vi "gcn_directory_monitor.vi"() -> ()   [LabVIEW 2017]
doc: "This example shows how we can use directory change notifications within the Windows API to monitor a folder for a change in a certain directory. We utilize the FindFirstChangeNotification to set up our events to monitor. We then utilize the wait functions to trigger a LV event when a change has been made to the directory. For more information on the Windows API, visit the MSDN."
panel:
  in  "browser_link":path
  in  "WebBrowser":refnum<k7>(container)
  in  "Stop Button":bool
  in  "Added?":string
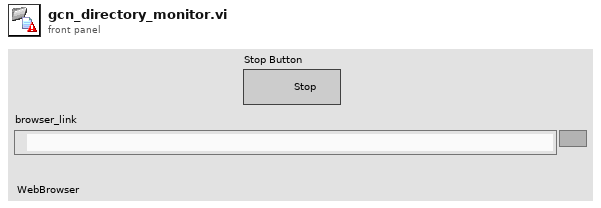
[diagram p1: front panel]
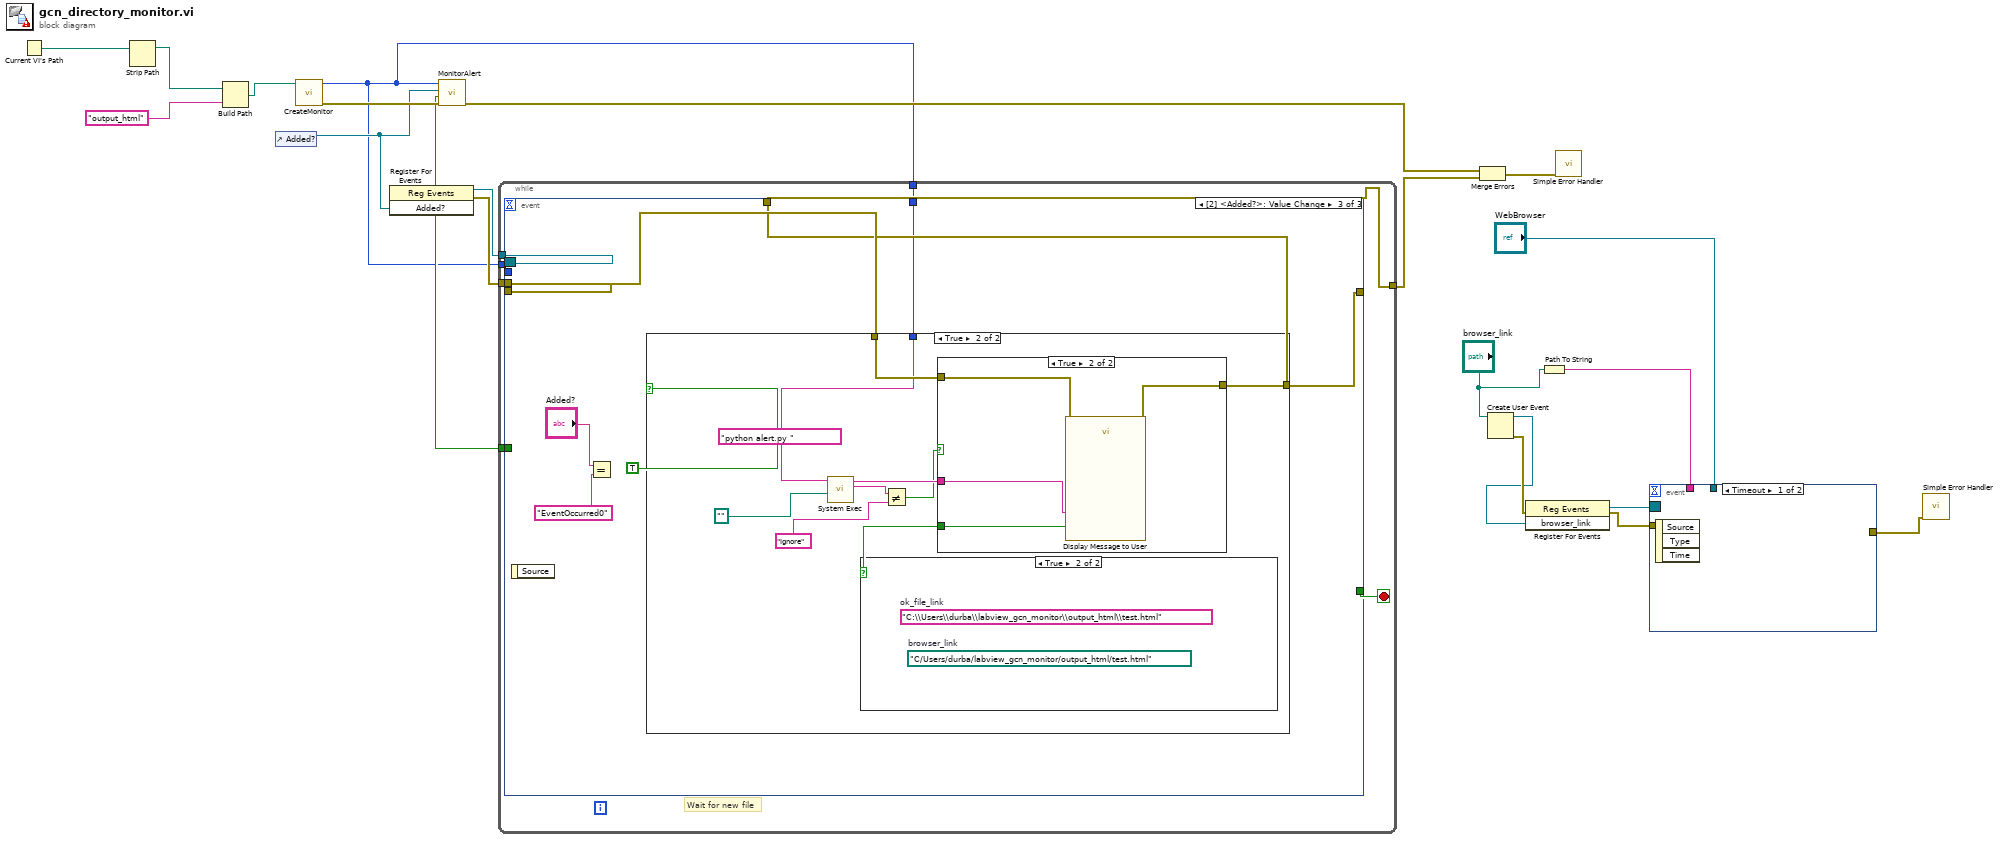
[diagram p0: block diagram]
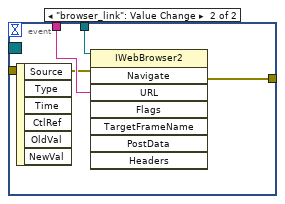
[diagram p2: hidden frame]
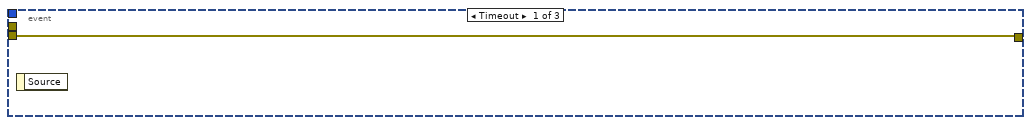
[diagram p3: hidden frame]
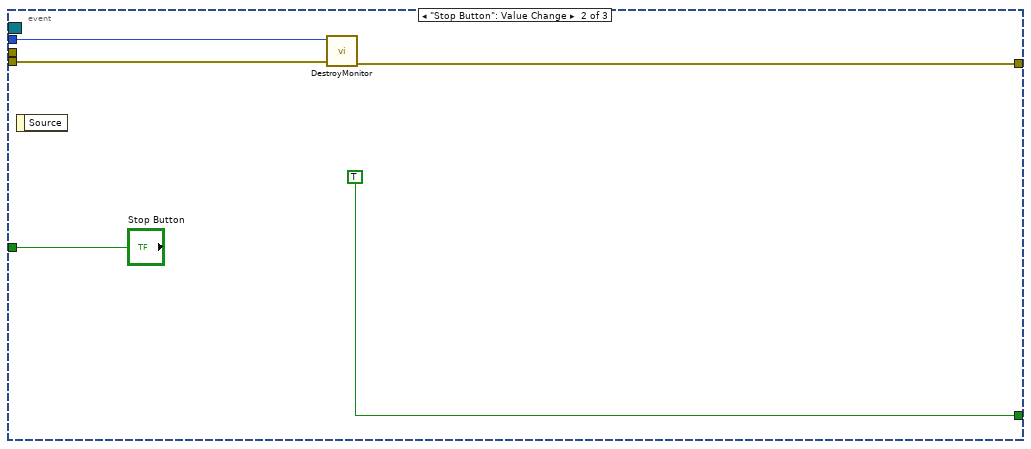
[diagram p4: hidden frame]
diagram:
  n1 = Current VI's Path() -> (path=w19:path)
  n2 = Strip Path(path=w19) -> (stripped path=w18:path)  [unwired: 1 out]
  n3 = Build Path(base path=w18, name or relative path="output_html") -> (appended path=w17:path)
  n4 = control-ref of="Added?"() -> (w20:refnum<vi>)
  n5 = call "CreateMonitor.vi"("File Path Control"=w17) -> ("error out"=w21:errorcluster, "Handle"=w1:i32)  [unwired: 9 in]
  n6 = register-events(w20) -> (reference out=w11:refnum<event-registration>, error out=w12:errorcluster)  [unwired: 2 in]
  n7 = while {
    tunnel: w1 -> [w27]
    tunnel: w11 -> [w26]
    tunnel: [w24] -> w14
    tunnel: w12 -> [w25]
    tunnel: [w23] -> w2
    tunnel: w1 -> [w22]
    stop <- w28 stop-if-true
    # "Wait for new file"
    n8 = event shown="[2] <Added?>: Value Change" {
      selector: w26 -> [_ _ _]
      dyn-events: _ -> [_ _ _]
      timeout: _ -> [_ _ _]
      tunnel: [_ TRUE _] -> w28
      tunnel: w27 -> [_ w34 _]
      tunnel: [w29 w32 w37] -> _
      tunnel: w25 -> [w29 w31 _]
      tunnel: w25 -> [_ _ w40]
      tunnel: [_ _ w37] -> w24
      tunnel: [_ "Stop Button" _] -> w23
      tunnel: w22 -> [_ _ w35]
      event Timeout {
        n9 = event-data() -> ()  [unwired: 1 in, 1 out]
      }
      event "Stop Button": Value Change {
        n10 = event-data() -> ()  [unwired: 1 in, 1 out]
        n11 = call "DestroyMonitor.vi"("Error In"=w31, "Handle in"=w34) -> ("Error Out"=w32:errorcluster)  [unwired: 9 in]
      }
      event Value Change {
        n12 = event-data() -> ()  [unwired: 1 in, 1 out]
        n13 = Equal?(x="Added?", y="EventOccurred0") -> ()  [unwired: 1 out]
        n14 = case shown="True" TRUE {
          tunnel: w40 -> [w41 w50]
          tunnel: [w41 w49] -> w37
          tunnel: w35 -> [_ w46]
          frame False {
          }
          frame True {
            w46 = "python alert.py "
            n15 = call <vilib>:"System Exec.vi"("working directory"=path "", "command line"=w46) -> ("standard error"=w43:string, "standard output"=w45:string)  [unwired: 6 in, 2 out]
            n16 = Not Equal?(x=w43, y="Ignore") -> (x != y?=w42:bool)
            n17 = case shown="True" w42 {
              tunnel: w50 -> [_ w54]
              tunnel: [_ w53] -> w49
              tunnel: [_ w52] -> w48
              tunnel: w45 -> [_ w51]
              frame False {
              }
              frame True {
                n18 = call "Display Message to User"("error in (no error)"=w54, "Message"=w51) -> ("error out"=w53:errorcluster, "OK"=w52:bool)  [unwired: 8 in]
              }
            }
            n19 = case shown="True" w48 {
              frame False {
              }
              frame True {
                (unwired) path "C:/Users/durba/labview_gcn_monitor/output_html/test.html"  # browser_link
                (unwired) "C:\\Users\\durba\\labview_gcn_monitor\\output_html\\test.html"  # ok_file_link
              }
            }
          }
        }
      }
    }
  }
  n20 = call "MonitorAlert.vi"("error in (no error)"=w21, "STOP"=w2, "Str Refnum"=w20, "Handle"=w1) -> ("error out"=w15:errorcluster)  [unwired: 7 in]
  n21 = Merge Errors "Merge Errors"(w15, w14) -> (w13:errorcluster)
  n22 = Create User Event(user event datatype="browser_link") -> (user event=w5:refnum<user-event>, error out=w8:errorcluster)  [unwired: 1 in]
  n23 = register-events(error in=w8, w5) -> (reference out=w6:refnum<event-registration>, error out=w9:errorcluster)  [unwired: 1 in]
  n24 = Path To String(path="browser_link") -> (string=w7:string)
  n25 = call <vilib>:"Simple Error Handler.vi"("error in (no error)"=w13) -> ()  [unwired: 4 in, 5 out]
  n26 = event shown="[0] Timeout" {
    selector: w6 -> [_ _]
    dyn-events: _ -> [_ _]
    timeout: _ -> [_ _]
    tunnel: "WebBrowser" -> [_ w57]
    tunnel: w7 -> [_ w56]
    tunnel: [_ w55] -> w10
    tunnel: w9 -> [_ w55]
    event Timeout {
      n27 = event-data() -> ()  [unwired: 1 in, 3 out]
    }
    event "browser_link": Value Change {
      n28 = event-data() -> ()  [unwired: 1 in, 6 out]
      n29 = invoke class="IWebBrowser2" method="Navigate"(reference=w57, "URL"=w56) -> ()  [unwired: 6 in, 8 out]
    }
  }
  n30 = call <vilib>:"Simple Error Handler.vi"("error in (no error)"=w10) -> ()  [unwired: 4 in, 5 out]
